vi "Increment Progress Bar.vi"(8 "error in (no error)":errorcluster, 9 "Step Number (0: inc)":i32, 10 "Step Name (\"\")":string, 11 "Progress Bar Dialog in":refnum<class "Loading Dialog.lvclass">) -> (0 "error out":errorcluster, 2 "Cancelled?":bool, 3 "Progress Bar Dialog out":refnum<class "Loading Dialog.lvclass">)   [LabVIEW 2020, in "VI Properties Editor.lvlib" / "Loading Dialog.lvclass"]
doc: "Calling this function will increment the progress bar by one. The optional input for 'Step Name' allows you to display text for the current item."
uses:
  Loading Dialog.lvclass
  Loading Dialog.lvclass/Loading Dialog.ctl
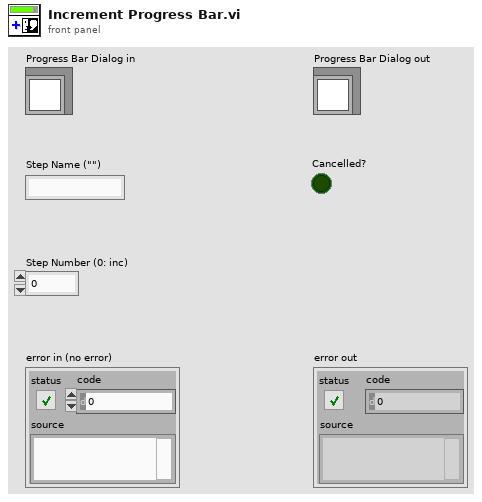
[diagram p1: front panel]
types:
  T1 = cluster{"Step Name (\"\")":string, "Step Number (0: inc)":i32}
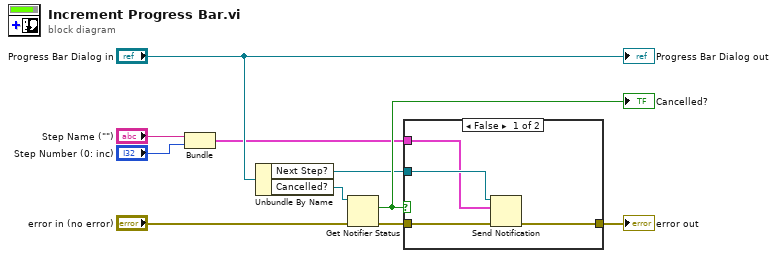
[diagram p0: block diagram]
diagram:
  n1 = Bundle("Step Name (\"\")"="Step Name (\"\")", "Step Number (0: inc)"="Step Number (0: inc)") -> (w1:T1)  [unwired: 1 in]
  n2 = Unbundle By Name("Progress Bar Dialog in") -> ("Next Step?"=w4:refnum<notifier>, "Cancelled?"=w9:refnum<notifier>)
  n3 = Get Notifier Status(notifier=w9, error in (no error)="error in (no error)") -> (current notification=w8:bool, error out=w6:errorcluster)  [unwired: 3 out]
  "Cancelled?" <- w8
  n4 = case shown="False" w8 {
    tunnel: w4 -> [w14 _]
    tunnel: w6 -> [w13 w15]
    tunnel: [w12 w15] -> w5
    tunnel: w1 -> [w11 _]
    frame False {
      n5 = Send Notification(notification=w11, notifier=w14, error in (no error)=w13) -> (error out=w12:errorcluster)  [unwired: 1 out]
    }
    frame True {
    }
  }
  "error out" <- w5
  "Progress Bar Dialog out" <- "Progress Bar Dialog in"
